vi "Start Pattern.vi"(8 "error in (no error)":errorcluster, 9 "Timeout":i32, 10 "Start Address":i32, 11 "CS++PPG in":refnum<class "CS++PPG.lvclass">) -> (0 "error out":errorcluster, 3 "CS++PPG out":refnum<class "CS++PPG.lvclass">)   [LabVIEW 2015, in "CS++PPG.lvlib" / "CS++PPG.lvclass"]
doc: "This VI starts the execution of the pattern (depending on the settings this could mean that the device first waits for an hardware trigger)."
uses:
  CS++PPG.lvclass
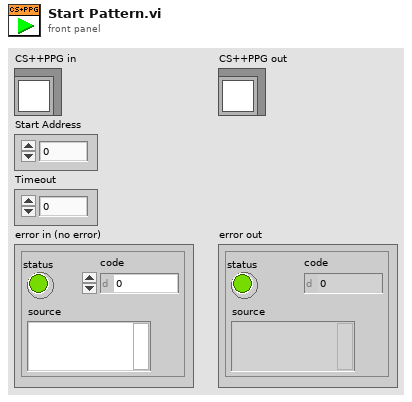
[diagram p1: front panel]
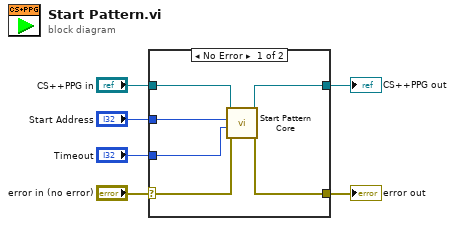
[diagram p0: block diagram]
diagram:
  n1 = case shown="No Error" "error in (no error)" {
    selector: "error in (no error)" -> [w10 w14]
    tunnel: [w9 w14] -> w5
    tunnel: [w11 w13] -> w3
    tunnel: "CS++PPG in" -> [w12 w13]
    tunnel: "Start Address" -> [w8 _]
    tunnel: "Timeout" -> [w7 _]
    frame No Error {
      n2 = call-dynamic "Start Pattern Core.vi"("error in (no error)"=w10, "Timeout"=w7, "Start Address"=w8, "CS++PPG in"=w12) -> ("error out"=w9:errorcluster, "CS++PPG out"=w11:refnum<class "CS++PPG.lvclass">)  [unwired: 6 in]
    }
    frame Error {
    }
  }
  "error out" <- w5
  "CS++PPG out" <- w3
